vi "DHE_DO_IMREAD_SHM.vi"(8 "error in":errorcluster) -> (0 "error out":errorcluster, 2 "response":string)   [LabVIEW 2016]
uses:
  Common/public/vis/CMN_FVAR_action.ctl
  SDSU_GBLVariables.vi
  DBSHAND/private/vis/DatabaseHand_Element_Get(string).vi
  DBSHAND/private/vis/DatabaseHand_Element_Get(I32).vi
  c/lib/libarcDHE.so
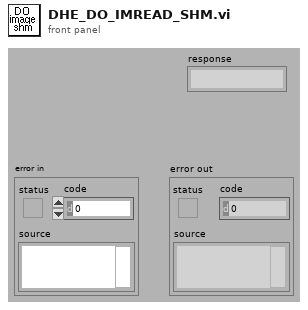
[diagram p1: front panel]
types:
  T1 = typedef "DatabaseHand_RefNum.ctl" = refnum<vi>
  T2 = enum16{"Idle", "Exposing", "Paused", "AbortExp", "Reading", "AbortRead", "FinishedReading", "Resetting", "Reducing"}
  T3 = cluster{"Video Processor Type":string, "support gain":bool, "Timing Board":string, "support reset":bool, "Utility Board":string, "Shutter":string, "Temperature":string, "support temp control":bool, "Detector Type":string, "Support MPP":string, "Support Binning":string, "Readout Mode":string, "support shutter control":bool}
  T4 = typedef "CMN_FVAR_action.ctl" = enum16{"read", "write"}
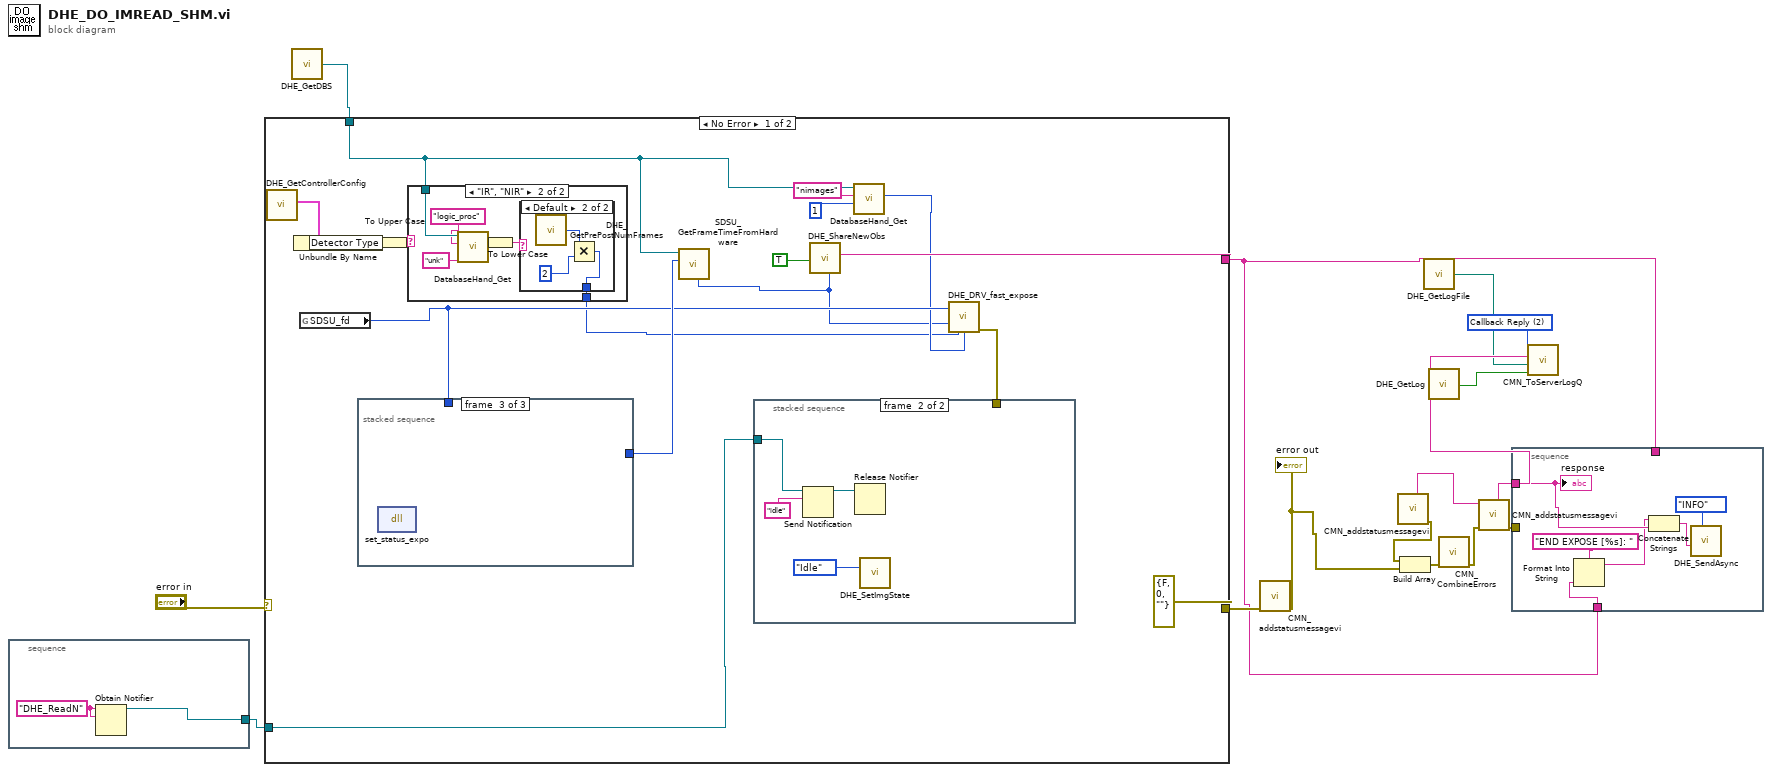
[diagram p0: block diagram]
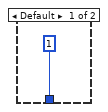
[diagram p2: hidden frame]
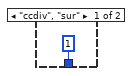
[diagram p3: hidden frame]
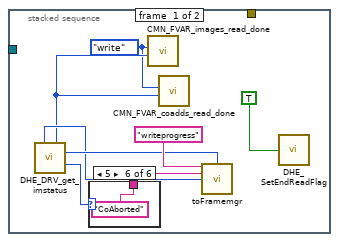
[diagram p4: hidden frame]
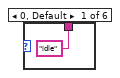
[diagram p5: hidden frame]
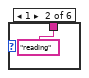
[diagram p6: hidden frame]
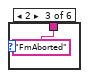
[diagram p7: hidden frame]
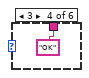
[diagram p8: hidden frame]
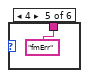
[diagram p9: hidden frame]
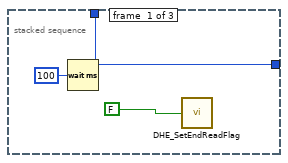
[diagram p10: hidden frame]
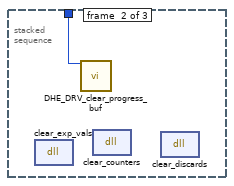
[diagram p11: hidden frame]
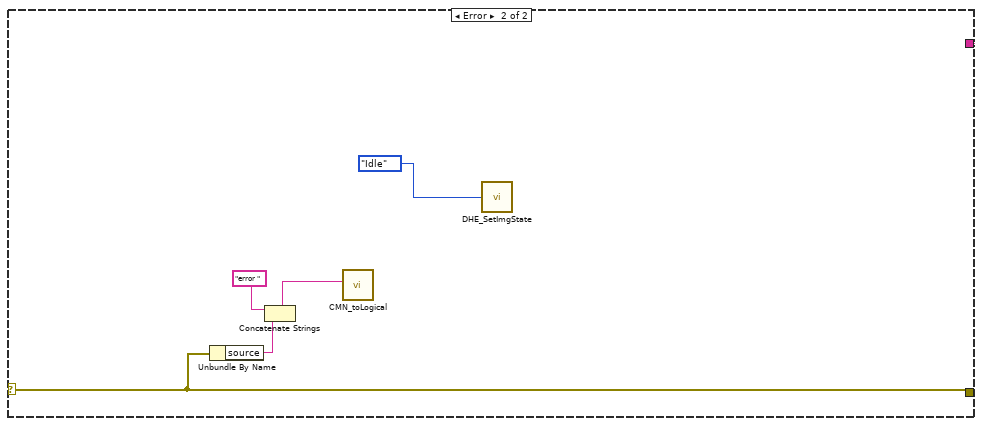
[diagram p12: hidden frame]
diagram:
  w14 = u16 2 items=["command", "imediateReply", "Callback Reply", "Information"] ("type")
  n1 = stacked-sequence {
    tunnel: [w16] -> w6
    frame #0 {
      w17 = "DHE_ReadN" ("name (unnamed)")
      n2 = Obtain Notifier(name (unnamed)=w17, notification data type=w17) -> (notifier out=w16:refnum<notifier>)  [unwired: 2 in, 2 out]
    }
  }
  n3 = call "DHE_GetDBS.vi"() -> ("DHE_DBSRef"=w3:T1)  [unwired: 9 out]
  n4 = case shown="No Error" "error in" {
    selector: "error in" -> [_ w71]
    tunnel: [errorcluster {"status"=FALSE, "code"=0, "source"=""} ("error IO") w71] -> w13
    tunnel: w3 -> [w19 _]
    tunnel: w6 -> [w27 _]
    tunnel: [w31 "" ("obsID")] -> w1
    frame No Error {
      n5 = call "DHE_GetControllerConfig.vi"() -> ("ControllerConfigCluster"=w30:T3)  [unwired: 11 out]
      n6 = Unbundle By Name(w30) -> ("Detector Type"=w29:string)
      n7 = global read "SDSU_GBLVariables.vi" "SDSU_fd"() -> (w24:i32)
      n8 = stacked-sequence {
        tunnel: w24 -> [w63 w66 _]
        tunnel: [w63 _ _] -> w33
        frame #0 {
          n9 = Wait (ms)(milliseconds to wait=u32 100) -> ()  [unwired: 1 out]
          n10 = call "DHE_SetEndReadFlag.vi"("DHE_read_ended"=FALSE ("readout ended")) -> ()  [unwired: 9 out]
        }
        frame #1 {
          n11 = dll-call lib="home/simager/panview/PAN/Modules/SDSU/private/c/lib/libarcDHE.so" fn="clear_exp_vals"() -> ()  [unwired: 3 in, 3 out]
          n12 = call "DHE_DRV_clear_progress_buf.vi"("fd"=w66) -> ()  [unwired: 1 in, 14 out]
          n13 = dll-call lib="home/simager/panview/PAN/Modules/SDSU/private/c/lib/libarcDHE.so" fn="clear_counters"() -> ()  [unwired: 3 in, 3 out]
          n14 = dll-call lib="home/simager/panview/PAN/Modules/SDSU/private/c/lib/libarcDHE.so" fn="clear_discards"() -> ()  [unwired: 3 in, 3 out]
        }
        frame #2 {
          n15 = dll-call lib="home/simager/panview/PAN/Modules/SDSU/private/c/lib/libarcDHE.so" fn="set_status_expo"() -> ()  [unwired: 3 in, 3 out]
        }
      }
      n16 = To Upper Case(1:w29) -> (0:w28:string)
      n17 = case shown="\"IR\", \"NIR\"" w28 {
        tunnel: [1 ("SDSU_fd") w40] -> w21
        tunnel: w19 -> [_ w36]
        frame Default {
        }
        frame "IR", "NIR" {
          n18 = call-poly "DatabaseHand_Get.vi"("default value"="unk", "name"="logic_proc", "Database RefNum in"=w36) -> ("value"=w38:string)  [unwired: 2 in, 6 out]
          n19 = To Lower Case(string=w38) -> (all lower case string=w37:string)
          n20 = case shown="Default" w37 {
            tunnel: [1 w42] -> w40
            frame "ccdiv", "sur" {
            }
            frame Default {
              n21 = call "DHE_GetPrePostNumFrames.vi"() -> ("DHE_PreExpose"=w44:i32)  [unwired: 9 out]
              n22 = Multiply(x=w44, y=2 ("SDSU_fd")) -> (x*y=w42:i32)
            }
          }
        }
      }
      n23 = call "SDSU_GetFrameTimeFromHardware.vi"("fd"=w33, "Database Ref"=w19) -> ("idle time"=w20:u32)  [unwired: 1 in, 8 out]
      n24 = call "DHE_ShareNewObs.vi"("exptime (ms)"=w20, "async?"=TRUE) -> ("obsID"=w31:string)  [unwired: 1 in, 8 out]
      n25 = call-poly "DatabaseHand_Get.vi"("default value"=1, "name"="nimages", "Database RefNum in"=w19) -> ("value"=w23:i32)  [unwired: 2 in, 6 out]
      n26 = call "DHE_DRV_fast_expose.vi"("fd"=w24, "expt_time"=w20, "frames_per_image"=w21, "nimages"=w23) -> ("error out"=w18:errorcluster)  [unwired: 2 in, 9 out]
      n27 = stacked-sequence {
        tunnel: w27 -> [_ w59]
        tunnel: w18 -> [_ _]
        frame #0 {
          w45 = CMN_FVAR_action."write" ("action")
          n28 = call "DHE_DRV_get_imstatus.vi"() -> ("ptr to buffer"=w48:u64, "buff read"=w49:i32, "frame status"=w51:i32, "images done"=w46:i32)  [unwired: 2 in, 10 out]
          n29 = case shown="5" w51 {
            tunnel: ["idle" "reading" "FmAborted" "OK" "fmErr" "CoAborted"] -> w50
            frame 0, Default {
            }
            frame 1 {
            }
            frame 2 {
            }
            frame 3 {
            }
            frame 4 {
            }
            frame 5 {
            }
          }
          n30 = call "CMN_FVAR_images_read_done.vi"("value in"=w46, "action"=w45) -> ()  [unwired: 9 out]
          n31 = call "CMN_FVAR_coadds_read_done.vi"("value in"=w46, "action"=w45) -> ()  [unwired: 9 out]
          n32 = call "toFramemgr.vi"("command"="writeprogress", "progress"=w49, "arg"=w50, "bufpointer"=w48) -> ()  [unwired: 5 in, 7 out]
          n33 = call "DHE_SetEndReadFlag.vi"("DHE_read_ended"=TRUE ("readout ended")) -> ()  [unwired: 9 out]
        }
        frame #1 {
          n34 = Send Notification(notification="idle", notifier=w59) -> (notifier out=w62:refnum<notifier>)  [unwired: 1 in, 1 out]
          n35 = Release Notifier(notifier=w62) -> ()  [unwired: 1 in, 4 out]
          n36 = call "DHE_SetImgState.vi"("DHE_ImgState"=T2."Idle" ("ImgState")) -> ()  [unwired: 9 out]
        }
      }
    }
    frame Error {
      n37 = Unbundle By Name(w71) -> ("source"=w70:string)
      n38 = Concatenate Strings("error " ("command"), w70) -> (w69:string)
      n39 = call "CMN_toLogical.vi"("command"=w69) -> ()  [unwired: 10 out]
      n40 = call "DHE_SetImgState.vi"("DHE_ImgState"=T2."Idle" ("ImgState")) -> ()  [unwired: 9 out]
    }
  }
  n41 = call "CMN_addstatusmessagevi.vi"("error in (no error)"=w13) -> ("error out"=w8:errorcluster)  [unwired: 1 in, 9 out]
  "error out" <- w8
  n42 = call "CMN_addstatusmessagevi.vi"() -> ("error out"=w9:errorcluster, "modified message out"=w7:string)  [unwired: 2 in, 8 out]
  n43 = Build Array(w9, w8) -> (w12:errorcluster[])
  n44 = call "DHE_GetLogFile.vi"() -> ("DHE_LogFile"=w4:path)  [unwired: 9 out]
  n45 = call "DHE_GetLog.vi"() -> ("DHE_log"=w5:bool)  [unwired: 9 out]
  n46 = call "CMN_CombineErrors.vi"("Errors"=w12) -> ("error out"=w11:errorcluster)  [unwired: 10 out]
  n47 = call "CMN_addstatusmessagevi.vi"("error in (no error)"=w11, "message  in"=w7) -> ("error out"=w2:errorcluster, "modified message out"=w10:string)  [unwired: 8 out]
  n48 = stacked-sequence {
    tunnel: w10 -> [w77]
    tunnel: w2 -> [_]
    tunnel: w1 -> [_]
    tunnel: w1 -> [w75]
    frame #0 {
      n49 = Format Into String(format string="END EXPOSE [%s]: " ("string"), w75) -> (resulting string=w74:string)  [unwired: 2 in, 1 out]
      n50 = Concatenate Strings(w74, w77) -> (w73:string)
      n51 = call "DHE_SendAsync.vi"("type"=enum16{"ERROR", "WARNING", "INFO", "CHANGED"}."INFO", "Message"=w73) -> ()  [unwired: 2 in, 8 out]
      "response" <- w77
    }
  }
  n52 = call "CMN_ToServerLogQ.vi"("Log"=w5, "file"=w4, "string"=w10, "type"=w14) -> ()  [unwired: 2 in, 5 out]
